vi "FPGA_read_test.vi"() -> ()   [LabVIEW 2013]
panel:
  out "output array":dbl[][](array[numeric]) format="%.2f"
  in  "milliseconds to wait":u32=100
  in  "Inst_parameter":T1={"Kind"=17, "Strings"=["ADC", "192.168.137.11", "V0;V1;V2;V3;V4;V5;V6;V7;V8;V9;V10;V11;V12;V13;V14;V15;V16;V17;V18;V19;V20;V21;V22;V23;V24;V25;V26;V27;V28;V29;V30;V31", "V;V;V;V;V;V;V;V;V;V;V;V;V;V;V;V;V;V;V;V;V;V;V;V;V;V;V;V;V;V;V;V", "1.0;1.0;1.0;1.0;1.0;1.0;1.0;1.0;1.0;1.0;1.0;1.0;1.0;1.0;1.0;1.0;1.0;1.0;1.0;1.0;1.0;1.0;1.0;1.0;1.0;1.0;1.0;1.0;1.0;1.0;1.0;1.0", "0;1;2;3;4;5;6;7;8;9;10;11;12;13;14;15;16;17;18;19;20;21;22;23;24;25;26;27;28;29;30;31", "10;10;10;10;10;10;10;10;10;10;10;10;10;10;10;10;10;10;10;10;10;10;10;10;10;10;10;10;10;10;10;10", "DIFF;DIFF;DIFF;DIFF;DIFF;DIFF;DIFF;DIFF;DIFF;DIFF;DIFF;DIFF;DIFF;DIFF;DIFF;DIFF;DIFF;DIFF;DIFF;DIFF;DIFF;DIFF;DIFF;DIFF;DIFF;DIFF;DIFF;DIFF;DIFF;DIFF;DIFF;DIFF"], "uint64s"=[32, 250000, 250, 0, 0, 2, 1], "Doubles"=[1.0], "DAQmx take out list"=[]}
  in  "DAC param":T2={"IP Adress FPGA"="192.168.137.11", "Delay(ms)"=1, "Busses to use"=[TRUE, TRUE, TRUE, FALSE, FALSE, FALSE, FALSE, FALSE], "max"=1.0, "min"=-1.0}
  in  "Stop":bool
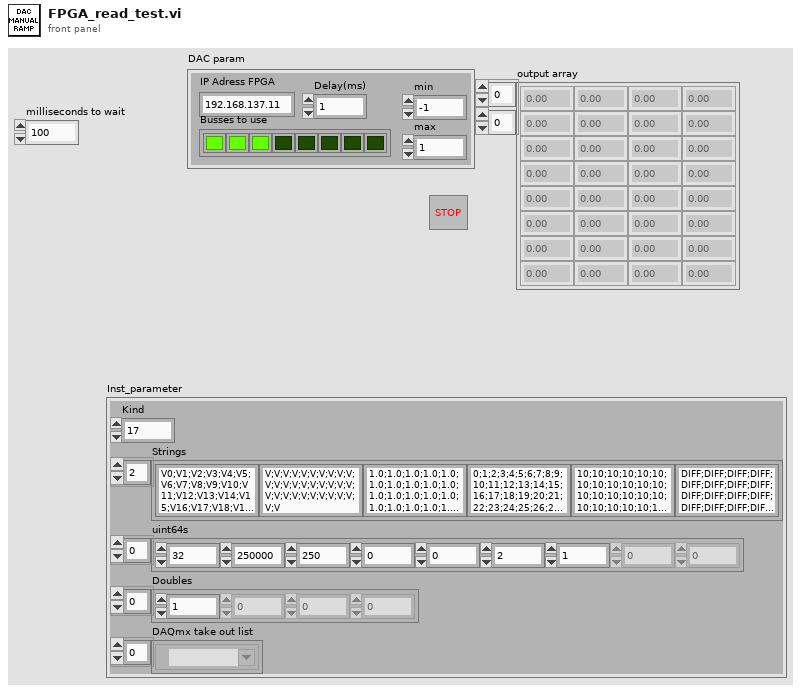
[diagram p1: front panel]
types:
  T1 = cluster{"Kind":u16, "Strings":string[], "uint64s":u64[], "Doubles":dbl[], "DAQmx take out list":refnum<k21>[]}
  T2 = cluster{"IP Adress FPGA":string, "Delay(ms)":u8, "Busses to use":bool[], "max":dbl, "min":dbl}
  T3 = enum8{"start movement", "buses to use", "delay", "value", "stop", ""}
  T4 = typedef "fpga-bitfile-ref.ctl" = refnum<k20>
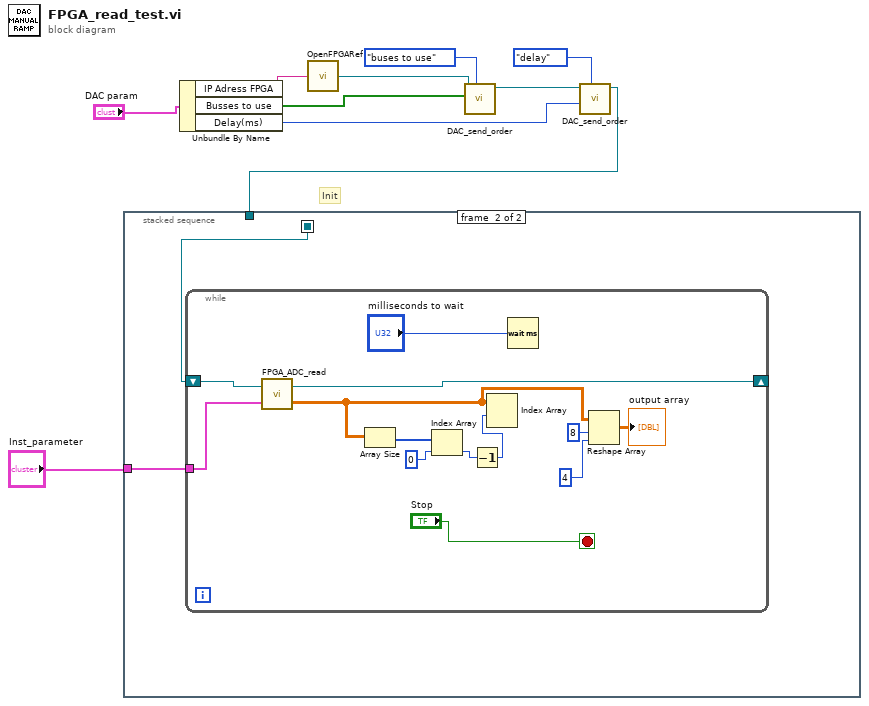
[diagram p0: block diagram]
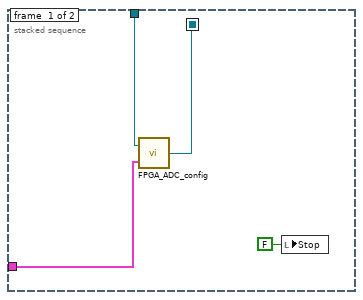
[diagram p2: hidden frame]
diagram:
  # "Init"
  n1 = Unbundle By Name("DAC param") -> ("IP Adress FPGA"=w6:string, "Busses to use"=w5:bool[], "Delay(ms)"=w4:u8)
  n2 = call "OpenFPGARef.vi"("IP Address"=w6) -> ("FPGA VI Reference Out"=w7:T4)
  n3 = call "DAC_send_order.vi"("order"=T3."buses to use", "buses to use"=w5, "FPGA VI Reference In"=w7) -> ("FPGA VI Reference Out"=w8:T4)  [unwired: 8 in]
  n4 = call "DAC_send_order.vi"("order"=T3."delay", "delay between steps (ms)"=w4, "FPGA VI Reference In"=w8) -> ("FPGA VI Reference Out"=w2:T4)  [unwired: 8 in]
  n5 = stacked-sequence {
    seq-local: [w12 _] -> [_ w16]
    tunnel: "Inst_parameter" -> [w14 w15]
    tunnel: w2 -> [w13 _]
    frame #0 {
      n6 = call "FPGA_ADC_config.vi"("Inst_parameter"=w14, "FPGA ref in"=w13) -> ("FPGA ref out"=w12:T4)
      n7 = local write "Stop"(FALSE ("Stop")) -> ()
    }
    frame #1 {
      n8 = while {
        shift-right: [w28] -> _
        shift-left: w16 -> [w29]
        tunnel: w15 -> [w27]
        stop <- "Stop" stop-if-true
        n9 = call "FPGA_ADC_read.vi"("Readout parameter"=w27, "FPGA In"=w29) -> ("data out"=w20:dbl[][], "FPGA Out"=w28:T4)
        n10 = Array Size(array=w20) -> (size(s)=w26:i32[])
        n11 = Index Array(array=w26, index=0) -> (element=w24:i32)
        n12 = Decrement(x=w24) -> (x-1=w23:i32)
        n13 = Index Array(array=w20, index (row)=w23) -> ()  [unwired: 1 in, 1 out]
        n14 = Wait (ms)(milliseconds to wait="milliseconds to wait") -> ()  [unwired: 1 out]
        n15 = Reshape Array(w20, 8 ("dimension size"), 4 ("dimension size")) -> (→"output array":dbl[][])
      }
    }
  }
